vi "Check for Cloned VI Name.vi"(3 "Possible Clone VI Name":string) -> (0 "Root VI Name":string)   [LabVIEW 2011]
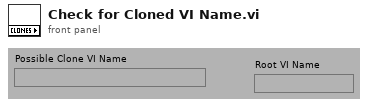
[diagram p1: front panel]
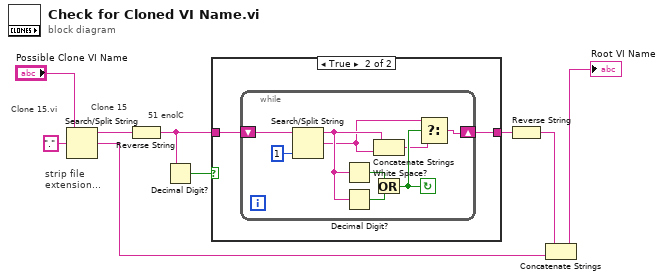
[diagram p0: block diagram]
diagram:
  # "strip file\nextension..."
  # "51 enolC"
  # "Clone 15"
  # "Clone 15.vi"
  n1 = Search/Split String(string="Possible Clone VI Name", search string/char (-)=".") -> (substring before match=w9:string, match + rest of string=w3:string)  [unwired: 2 out]
  n2 = Reverse String(1:w9) -> (0:w2:string)
  n3 = Decimal Digit?(1:w2) -> (0:w1:bool)
  n4 = case shown="True" w1 {
    tunnel: [w10 w12] -> w5
    tunnel: w2 -> [w10 w11]
    frame False {
    }
    frame True {
      n5 = while {
        shift-right: [w14] -> w12
        shift-left: w11 -> [w21]
        stop <- w17 continue-if-true
        n6 = Search/Split String(string=w21, offset (0)=1) -> (substring before match=w16:string, match + rest of string=w13:string)  [unwired: 2 out]
        n7 = White Space?(1:w16) -> (0:w18:bool)
        n8 = Decimal Digit?(1:w16) -> (0:w19:bool)
        n9 = Concatenate Strings(w16, w13) -> (w15:string)
        n10 = Or(x=w18, y=w19) -> (x .or. y?=w17:bool)
        n11 = Select(t=w13, s=w17, f=w15) -> (s? t:f=w14:string)
      }
    }
  }
  n12 = Reverse String(1:w5) -> (0:w4:string)
  n13 = Concatenate Strings(w4, w3) -> (→"Root VI Name":string)
